vi "Check_Particle_State_NextTime.vi"(0 "Particle State at T":T3(array[cluster]), 1 "Torque":bool, 2 "Torque":dbl, 5 "Tau_On":i32, 7 "Tau_Off":i32, 9 "Ini_Anchor_Posi":dbl[][](array[numeric]), 11 "Center State at T":T1, 12 "Asymmetry (X, Y)":dbl[](array[numeric]), 13 "SD":dbl) -> (4 "Particle State at T+1":T2(array[cluster]), 10 "Ini_Anchor_Posi":dbl[][](array[numeric]), 15 "New Center State at T":T1)   [LabVIEW 2014]
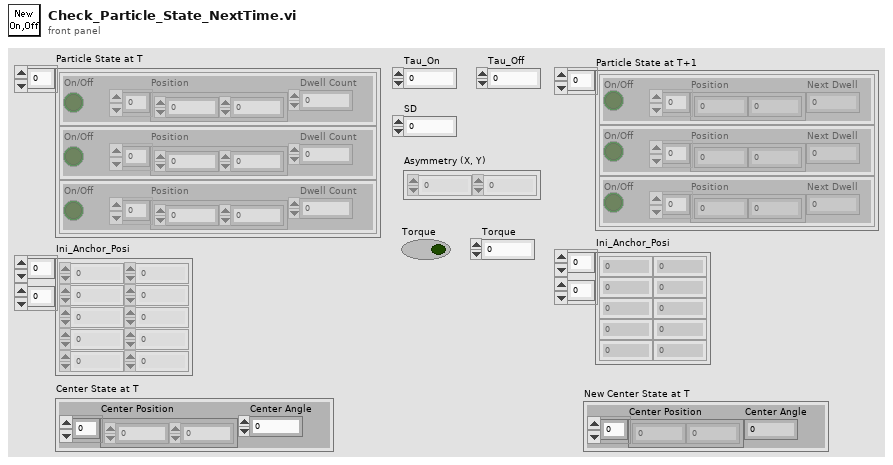
[diagram p1: front panel]
types:
  T1 = cluster{"Center Position":dbl[], "Center Angle":dbl}
  T2 = cluster{"On/Off":bool, "Position":dbl[], "Next Dwell":i32}[]
  T3 = cluster{"On/Off":bool, "Position":dbl[], "Dwell Count":i32}[]
  T4 = cluster{"On/Off":bool, "Position":dbl[], "Next Dwell":i32}
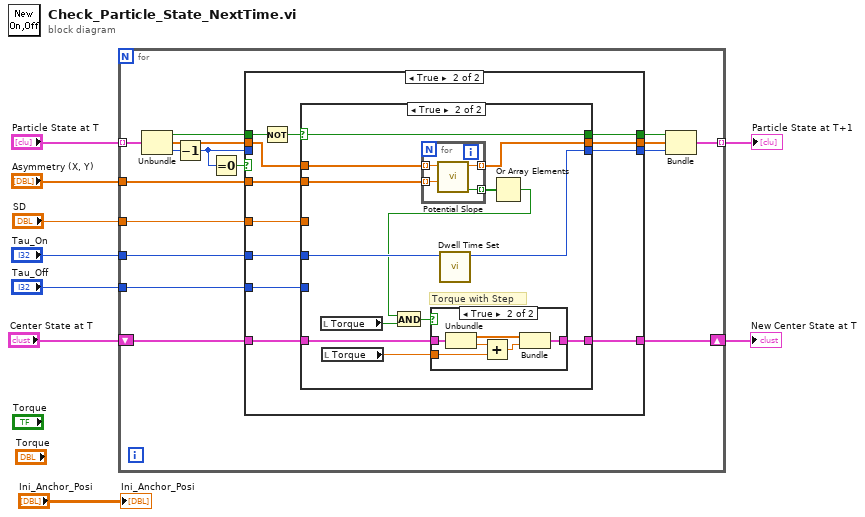
[diagram p0: block diagram]
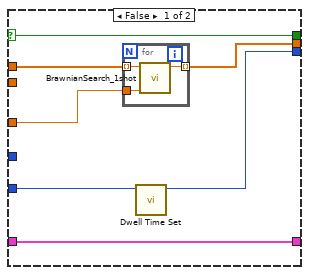
[diagram p3: hidden frame]
diagram:
  n1 = for {
    tunnel: "Particle State at T" -> [w25] mode=indexing
    tunnel: "Tau_On" -> [w18]
    tunnel: "Tau_Off" -> [w16]
    tunnel: [w15] -> w6 mode=indexing
    tunnel: "Asymmetry (X, Y)" -> [w13]
    tunnel: "SD" -> [w12]
    shift-right: [w10] -> w2
    shift-left: "Center State at T" -> [w11]
    n2 = Unbundle(w25) -> ("On/Off"=w22:bool, "Position"=w21:dbl[], "Dwell Count"=w24:i32)
    n3 = Decrement(x=w24) -> (x-1=w14:i32)
    n4 = Equal To 0?(x=w14) -> (x = 0?=w23:bool)
    n5 = case shown="True" w23 {
      tunnel: w22 -> [w29 w37]
      tunnel: [w29 w33] -> w20
      tunnel: w21 -> [w28 w36]
      tunnel: [w28 w34] -> w19
      tunnel: w18 -> [_ w41]
      tunnel: [w27 w40] -> w17
      tunnel: w16 -> [_ w39]
      tunnel: w14 -> [w27 _]
      tunnel: w13 -> [_ w35]
      tunnel: w12 -> [_ w32]
      tunnel: w11 -> [w26 w31]
      tunnel: [w26 w30] -> w10
      frame False {
      }
      frame True {
        n6 = Not(x=w37) -> (.not. x?=w38:bool)
        n7 = case shown="True" w38 {
          selector: w38 -> [w46 w60]
          tunnel: w41 -> [_ w64]
          tunnel: [w47 w63] -> w40
          tunnel: w39 -> [w48 _]
          tunnel: w36 -> [w45 w62]
          tunnel: w35 -> [_ w61]
          tunnel: [w44 w54] -> w34
          tunnel: [w46 w60] -> w33
          tunnel: w32 -> [w43 _]
          tunnel: w31 -> [w42 w59]
          tunnel: [w42 w58] -> w30
          frame False {
            n8 = for {
              tunnel: w45 -> [w51] mode=indexing
              tunnel: [w50] -> w44 mode=indexing
              tunnel: w43 -> [w49]
              n9 = call "BrawnianSearch_1shot.vi"("SD"=w49, "Start Position"=w51) -> ("Final Position"=w50:dbl)  [unwired: 9 in]
            }
            n10 = call "Dwell Time Set.vi"("Tau"=w48) -> ("Next Dwell"=w47:i32)  [unwired: 10 in]
          }
          frame True {
            # "Torque with Step"
            n11 = local read "Torque"() -> (w56:bool)
            n12 = local read "Torque"() -> (w57:dbl)
            n13 = for {
              tunnel: w62 -> [w75] mode=indexing
              tunnel: w61 -> [w74] mode=indexing
              tunnel: [w73] -> w54 mode=indexing
              tunnel: [w72] -> w53 mode=indexing
              n14 = call "Potential Slope.vi"("Asymmetry"=w74, "Position"=w75) -> ("Step"=w72:bool, "New Position"=w73:dbl)  [unwired: 7 in, 1 out]
            }
            n15 = call "Dwell Time Set.vi"("Tau"=w64) -> ("Next Dwell"=w63:i32)  [unwired: 10 in]
            n16 = Or Array Elements(Boolean array=w53) -> (logical OR=w52:bool)
            n17 = And(x=w52, y=w56) -> (x .and. y?=w55:bool)
            n18 = case shown="True" w55 {
              tunnel: w59 -> [w65 w71]
              tunnel: [w65 w69] -> w58
              tunnel: w57 -> [_ w66]
              frame False {
              }
              frame True {
                n19 = Unbundle(w71) -> ("Center Position"=w70:dbl[], "Center Angle"=w68:dbl)
                n20 = Add(x=w68, y=w66) -> (x+y=w67:dbl)
                n21 = Bundle("Center Position"=w70, w67) -> (w69:cluster{"Center Position":dbl[], dbl})  [unwired: 1 in]
              }
            }
          }
        }
      }
    }
    n22 = Bundle("On/Off"=w20, "Position"=w19, "Next Dwell"=w17) -> (w15:T4)  [unwired: 1 in]
  }
  "Particle State at T+1" <- w6
  "New Center State at T" <- w2
  "Ini_Anchor_Posi" <- "Ini_Anchor_Posi"
